vi "Set Top Level Library.vi"(8 "error in (no error)":errorcluster, 10 "ProjectItem Refnum":refnum<vi>, 11 "PPL in":refnum<class "NI_AB_API_PPL.lvclass">) -> (0 "error out":errorcluster, 3 "PPL out":refnum<class "NI_AB_API_PPL.lvclass">)   [LabVIEW 2020, in "NI_AB_API_PPL.lvclass"]
uses:
  <vilib>/AppBuilder/AB_API/PPL/NI_AB_API_PPL.lvclass
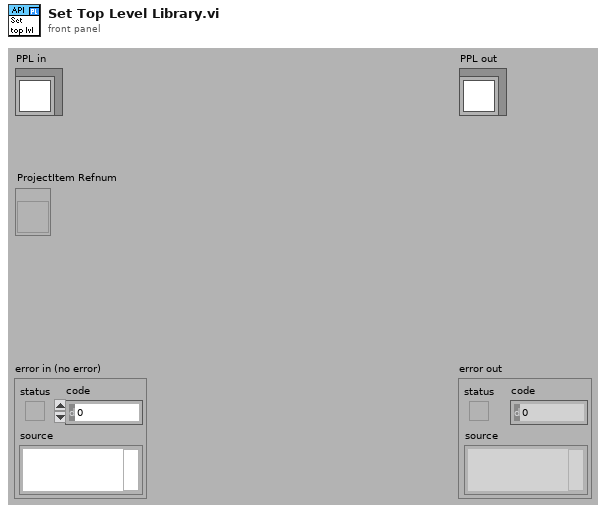
[diagram p1: front panel]
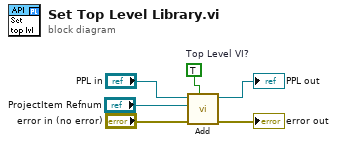
[diagram p0: block diagram]
diagram:
  w3 = TRUE  # Top Level VI?
  n1 = call-dynamic "Add.vi"("Top Level Library?"=w3, "error in (no error)"="error in (no error)", "ProjectItem Refnum"="ProjectItem Refnum", "PPL in"="PPL in") -> ("error out"=→"error out":errorcluster, "PPL out"=→"PPL out":refnum<class "NI_AB_API_PPL.lvclass">)  [unwired: 6 in]
